vi "TopLevelDiagram to Code.vi"(10 "C code":string, 11 "Diagram ref":refnum<vi>) -> (3 "transcripted code":string)   [LabVIEW 2018]
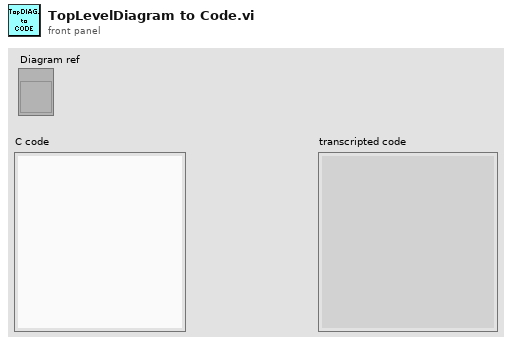
[diagram p1: front panel]
types:
  T1 = cluster{"wire labels":string[], "wire terminals datatypes":string[][]}
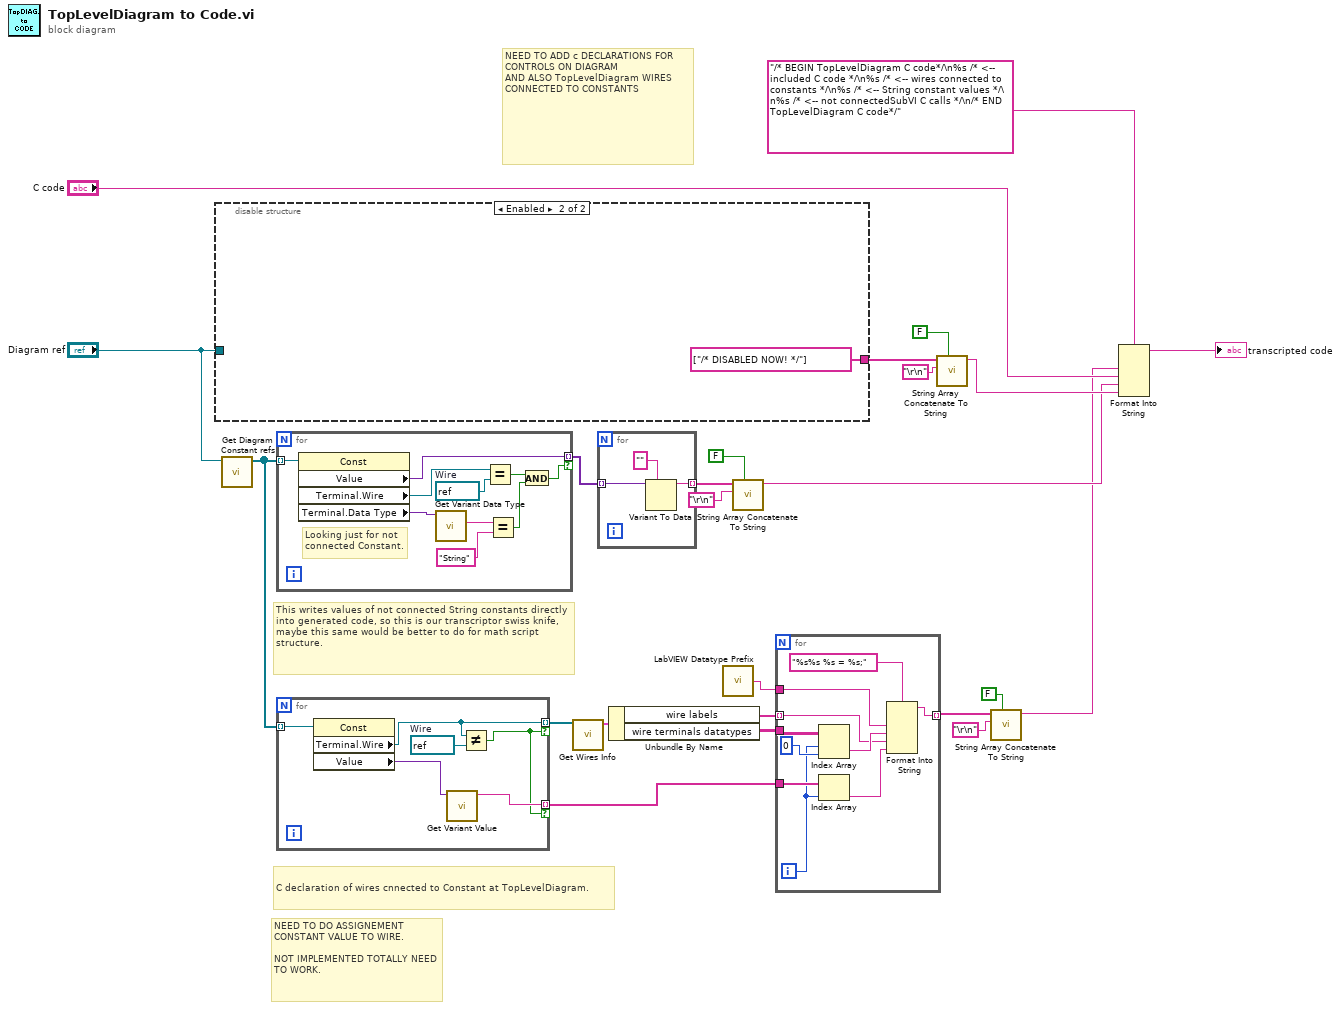
[diagram p0: block diagram]
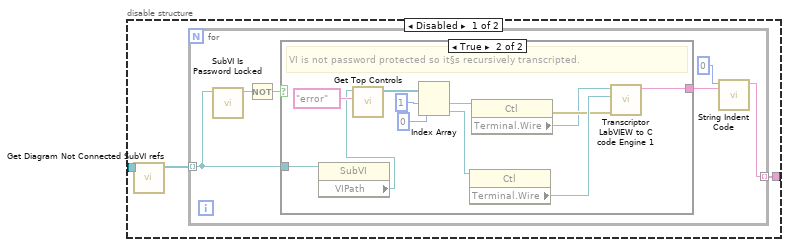
[diagram p2: hidden frame]
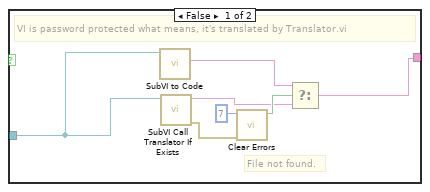
[diagram p3: hidden frame]
diagram:
  # "NEED TO DO ASSIGNEMENT CONSTANT VALUE TO WIRE.\n\nNOT IMPLEMENTED TOTALLY NEED TO WORK."
  # "C declaration of wires cnnected to Constant at TopLevelDiagram."
  # "NEED TO ADD c DECLARATIONS FOR CONTROLS ON DIAGRAM\nAND ALSO TopLevelDiagram WIRES CONNECTED TO CONSTANTS"
  # "This writes values of not connected String constants directly into generated code, so this is our transcriptor swiss knife, maybe this same would be better to do for math script structure."
  n1 = disable-structure shown="Enabled" {
    disable-tunnel: [w26 string[] ["/* DISABLED NOW! */"] ("Array String In")] -> w24
    disable-tunnel: "Diagram ref" -> [w25 _]
    frame Disabled {
      n2 = call "Get Diagram Not Connected SubVI refs.vi"("Diagram ref."=w25) -> ("not connected SubVIs[]"=w27:refnum<vi>[])  [unwired: 10 in]
      n3 = for {
        tunnel: w27 -> [w33] mode=indexing
        tunnel: [w28] -> w26 mode=indexing
        n4 = call "SubVI Is Password Locked.vi"("SubVI ref"=w33) -> ("isPasswordLocked?"=w32:bool)  [unwired: 9 in, 1 out]
        n5 = Not(x=w32) -> (.not. x?=w31:bool)
        n6 = case shown="True" w31 {
          tunnel: [w34 w42] -> w29
          tunnel: w33 -> [w36 w41]
          frame False {
            # "File not found."
            # "VI is password protected what means, it's translated by Translator.vi"
            n7 = call "SubVI to Code.vi"("reference"=w36) -> ("C code"=w35:string)  [unwired: 9 in, 1 out]
            n8 = call "SubVI Call Translator If Exists.vi"("SubVI Refnum"=w36) -> ("Error Out"=w37:errorcluster, "Replaced Code"=w39:string)  [unwired: 7 in, 2 out]
            n9 = call <vilib>:"Clear Errors.vi"("error in (no error)"=w37, "specific error code to clear (0: all)"=7) -> ("specific error cleared?"=w40:bool)  [unwired: 4 in, 1 out]
            n10 = Select(t=w35, s=w40, f=w39) -> (s? t:f=w34:string)
          }
          frame True {
            # "VI is not password protected so it§s recursively transcripted."
            n11 = property on="Property Node" class="SubVI"(reference=w41) -> ("VIPath"=w43:path)  [unwired: 1 in, 2 out]
            n12 = call "Get Top Controls.vi"("DataType"="error", "vi path"=w43) -> ("Controls Referencies Array"=w45:refnum<vi>[])  [unwired: 8 in, 1 out]
            n13 = Index Array(array=w45, index #1=1 ("index"), index #2=0 ("index")) -> (element #1=w46:refnum<vi>, element #2=w51:refnum<vi>)
            n14 = property on="Property Node" class="Ctl"(reference=w51) -> ("Terminal.Wire"=w52:refnum<vi>)  [unwired: 1 in, 2 out]
            n15 = property on="Property Node" class="Ctl"(reference=w46) -> (error out=w49:errorcluster, "Terminal.Wire"=w47:refnum<vi>)  [unwired: 1 in, 1 out]
            n16 = call "Transcriptor LabVIEW to C code Engine 1.vi"("error in (no error)"=w49, "GObject stop"=w52, "GObject start"=w47) -> ("Transcripted code"=w42:string)  [unwired: 7 in, 1 out]
          }
        }
        n17 = call "String Indent Code.vi"("complete code"=w29, "actual nested level"=0) -> ("indented code"=w28:string)  [unwired: 9 in]
      }
    }
    frame Enabled {
    }
  }
  n18 = call "Get Diagram Constant refs.vi"("Diagram ref."="Diagram ref") -> ("Constant"=w15:refnum<vi>[])  [unwired: 10 in]
  n19 = for {
    tunnel: w15 -> [w63] mode=indexing
    tunnel: [w57] -> w19 mode=indexing if=w56
    w62 = refnum<vi> refnum  # Wire
    # "Looking just for not connected Constant."
    n20 = property class="Const"(reference=w63) -> ("Value"=w57:variant, "Terminal.Wire"=w58:refnum<vi>, "Terminal.Data Type"=w59:variant)  [unwired: 1 in, 2 out]
    n21 = call "Get Variant Data Type.vi"("Variant in"=w59) -> ("first data type"=w61:string)  [unwired: 9 in, 1 out]
    n22 = Equal?(x=w58, y=w62) -> (x = y?=w55:bool)
    n23 = Equal?(x=w61, y="String") -> (x = y?=w54:bool)
    n24 = And(x=w55, y=w54) -> (x .and. y?=w56:bool)
  }
  n25 = for {
    tunnel: w15 -> [w69] mode=indexing
    tunnel: [w67] -> w14 mode=indexing if=w64
    tunnel: [w65] -> w7 mode=indexing if=w64
    w68 = refnum<vi> refnum  # Wire
    n26 = property class="Const"(reference=w69) -> ("Terminal.Wire"=w67:refnum<vi>, "Value"=w66:variant)  [unwired: 1 in, 2 out]
    n27 = call "Get Variant Value.vi"("Variant in"=w66) -> ("Variant value as string"=w65:string)  [unwired: 10 in]
    n28 = Not Equal?(x=w67, y=w68) -> (x != y?=w64:bool)
  }
  n29 = call "Get Wires Info.vi"("connected\nwires refs."=w14) -> ("wires info cluster"=w13:T1)  [unwired: 10 in]
  n30 = for {
    tunnel: w19 -> [w72] mode=indexing
    tunnel: [w70] -> w18 mode=indexing
    n31 = Variant To Data(type="", Variant=w72) -> (data=w70:string)  [unwired: 1 in, 1 out]
  }
  n32 = Unbundle By Name(w13) -> ("wire labels"=w12:string[], "wire terminals datatypes"=w11:string[][])
  n33 = call "LabVIEW Datatype Prefix.vi"() -> ("datatype prefix"=w8:string)
  n34 = call "String Array Concatenate To String.vi"("insert last delimiter?"=FALSE, "Delimiter char"="\r\n", "Array String In"=w18) -> ("String"=w16:string)  [unwired: 8 in]
  n35 = for {
    tunnel: w12 -> [w79] mode=indexing
    tunnel: w11 -> [w82]
    tunnel: [w77] -> w10 mode=indexing
    tunnel: w8 -> [w76]
    tunnel: w7 -> [w75]
    i -> [w74]
    n36 = Index Array(array=w82, index (row)=w74, index (col)=0 ("disabled index (col)")) -> (element=w81:string)
    n37 = Index Array(array=w75, index=w74) -> (element=w73:string)
    n38 = Format Into String(format string="%s%s %s = %s;", w76, w81, w79, w73) -> (resulting string=w77:string)  [unwired: 2 in, 1 out]
  }
  n39 = call "String Array Concatenate To String.vi"("insert last delimiter?"=FALSE, "Delimiter char"="\r\n", "Array String In"=w24) -> ("String"=w23:string)  [unwired: 8 in]
  n40 = call "String Array Concatenate To String.vi"("insert last delimiter?"=FALSE, "Delimiter char"="\r\n", "Array String In"=w10) -> ("String"=w9:string)  [unwired: 8 in]
  n41 = Format Into String(format string="/* BEGIN TopLevelDiagram C code*/\n%s /* <-- included C code */\n%s /* <-- wires connected to constants */\n%s /* <-- String constant values */\n%s /* <-- not connectedSubVI C calls */\n/* END TopLevelDiagram C code*/", w9, "C code", w16, w23) -> (resulting string=→"transcripted code":string)  [unwired: 2 in, 1 out]
